vi "Auto Balance Error Tolerance DAO.vi"(0 "Auto Balance Increment Actions":T4, 3 "Config Ref":T3, 5 "LBCB Number":T1, 7 "Auto Balance Error In":T2, 11 "error in (no error)":errorcluster) -> (8 "Auto Balance Error Out":T2, 14 "Config Ref  out":T3, 15 "error out":errorcluster)   [LabVIEW 2013]
uses:
  Metadata/Persistant DAO Actions.ctl
  Metadata/Actuator Point.ctl
  <vilib>/Utility/config.llb/Config Data RefNum.ctl
  Metadata/LBCB Number.ctl
  <vilib>/Utility/config.llb/NI_LVConfig.lvlib
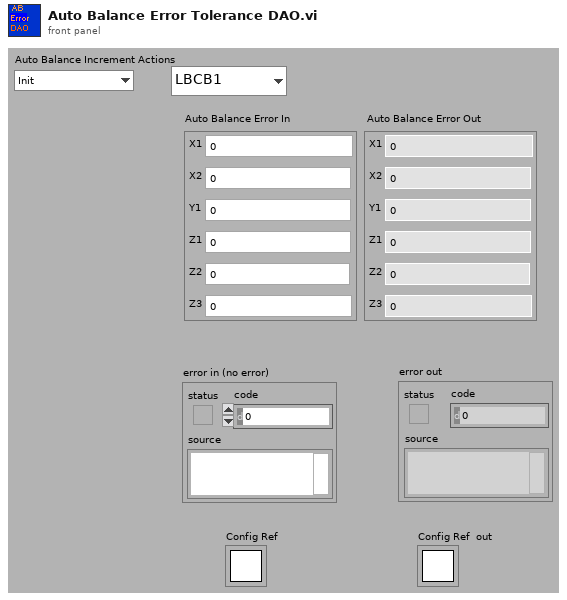
[diagram p1: front panel]
types:
  T1 = typedef "LBCB Number.ctl" = enum16{"LBCB1", "LBCB2"}
  T2 = typedef "Actuator Point.ctl" = cluster{"X1":dbl, "X2":dbl, "Y1":dbl, "Z1":dbl, "Z2":dbl, "Z3":dbl}
  T3 = typedef "NI_LVConfig.lvlib/Config Data RefNum.ctl" = refnum<k1>
  T4 = typedef "Persistant DAO Actions.ctl" = enum16{"Init", "Get", "Set", "Load", "Save"}
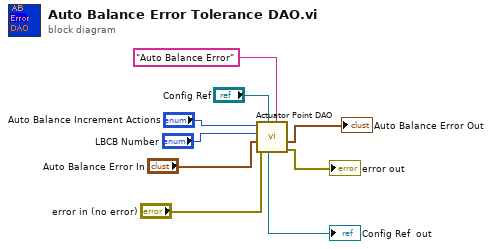
[diagram p0: block diagram]
diagram:
  n1 = call "Actuator Point DAO.vi"("section"="Auto Balance Error", "Config Ref  In"="Config Ref", "error in (no error)"="error in (no error)", "Point In"="Auto Balance Error In", "LBCB Number"="LBCB Number", "Actions"="Auto Balance Increment Actions") -> ("error out"=→"error out":errorcluster, "Point Out"=→"Auto Balance Error Out":T2, "Config Ref Out"=→"Config Ref  out":T3)  [unwired: 3 out]
